vi "Create GB 2014-11-10.vi"(6 "Edge Duplication Range":dbl=3.0, 7 "Skip cleanup if no subset":bool, 8 "Reduce to Repeating":T2={"Slab X"=4.0, "Slab Y"=4.0, "Tolerance (A)"=0.5, "Presorted?"=FALSE}, 9 "Min Seperation Distance (A)":dbl=1.5, 10 "Grain Growth and Geometry":T3={"Grain 1 Length (prop)"=1.0, "Grain 2 Length (prop)"=1.0, "Max Grain Height (A)"=80.0, "Max Grain Width (A)"=80.0, "Grain 1 Start"=-0.001, "Overlap Region (A)"=0.001}, 11 "Grain Boundary Definition":T4={"Grain 1 Orientation"=[1.0, 1.0, 1.0], "Grain 2 Orientation"=[1.0, 1.0, 1.0], "Twist Angle (Deg)"=60.0, "Translation Vector"=[0.0, 0.0, 0.0]}) -> (0 "GB Data":string[][](array[string]), 1 "Reduced Orthorhombic?":bool=TRUE, 2 "Reduced Monoclinic?":bool=TRUE, 3 "Grain Boundary":T5={"Structure Name"="(60.0) twist [1,1,1] [1,1,1+0.0tilt] (0.00,0.00,0.00)T GB", "Lattice vector a"=[2.339033413721388, 4.05132471316672, 0.0], "Lattice vector b"=[4.678066827442776, 0.0, 0.0], "Lattice vector c"=[0.0, 0.0, 46.0], "Atoms Array"=[{"Atom Name"="Cd", "Positions (Direct)"=[[0.00024683284377352164, 9.034709130927474e-05, -0.0008722454374929306], [0.0002468328437733024, 9.034709130938435e-05, 0.24912775456250708], [0.0002468328437733024, 9.034709130938435e-05, 0.49912775456250713], [0.33358016617710656, 0.33342368042464277, 0.08305707760779221], [0.33358016617710656, 0.33342368042464277, 0.3321630930398645], [0.6669134995104397, 0.6667570137579764, 0.41519843151722197], [0.6669134995104399, 0.6667570137579764, 0.16609241608514966], [0.00024683284377352164, 9.034709130927474e-05, 0.749127754562507], [0.33358016617710673, 0.33342368042464277, 0.6660924160851497], [0.33358016617710695, 0.33342368042464265, 0.9151984315172218], [0.6669134995104401, 0.6667570137579764, 0.5830570776077922], [0.6669134995104403, 0.6667570137579764, 0.8321630930398645]], "Positions (Cartesian)"=[[0.0, 8.881784197001252e-16, -0.04112329012467342], [0.0, 0.0, 11.458876709875327], [0.0, 0.0, 22.958876709875327], [2.339033413721388, 1.350441571055573, 3.819625569958442], [2.339033413721388, 1.350441571055573, 15.278502279833768], [4.678066827442776, 2.700883142111145, 19.09812784979221], [4.678066827442776, 2.700883142111146, 7.639251139916884], [0.0, 8.881784197001252e-16, 34.45887670987533], [2.3390334137213884, 1.3504415710555737, 30.639251139916883], [2.3390334137213884, 1.3504415710555746, 42.098127849792206], [4.678066827442777, 2.700883142111147, 26.819625569958443], [4.678066827442777, 2.700883142111148, 38.278502279833766]]}, {"Atom Name"="Te", "Positions (Direct)"=[[0.0002468328437733024, 9.034709130938435e-05, 0.062298242988452865], [0.0002468328437733024, 9.034709130938435e-05, 0.31140425842052516], [0.3335801661771065, 0.33342368042464277, 0.14533358146581032], [0.3335801661771065, 0.33342368042464277, 0.39443959689788266], [0.6669134995104397, 0.6667570137579764, 0.47747493537524005], [0.6669134995104399, 0.6667570137579764, 0.22836891994316774], [0.000246832843773325, 9.034709130937305e-05, 0.5622982429884529], [0.00024683284377354425, 9.034709130926343e-05, 0.811404258420525], [0.33358016617710684, 0.3334236804246426, 0.7283689199431677], [0.33358016617710706, 0.3334236804246425, 0.97747493537524], [0.6669134995104401, 0.6667570137579764, 0.6453335814658103], [0.6669134995104403, 0.6667570137579764, 0.8944395968978825]], "Positions (Cartesian)"=[[0.0, 0.0, 2.864719177468832], [0.0, 0.0, 14.323595887344158], [2.339033413721388, 1.3504415710555728, 6.684344747427275], [2.339033413721388, 1.3504415710555728, 18.1432214573026], [4.678066827442776, 2.700883142111145, 21.96284702726104], [4.678066827442776, 2.700883142111146, 10.503970317385717], [0.0, 9.181246808733296e-17, 25.86471917746883], [0.0, 9.799908877874582e-16, 37.323595887344155], [2.339033413721388, 1.3504415710555742, 33.503970317385715], [2.339033413721388, 1.350441571055575, 44.96284702726104], [4.678066827442777, 2.700883142111147, 29.684344747427275], [4.678066827442777, 2.700883142111148, 41.1432214573026]]}], "# of atoms"=24} {"Atoms Array"."Positions (Cartesian)" format="%#_4f"; "Atoms Array"."Positions (Direct)" format="%#_4f"}, 4 "Creation Time":T1={"Time to create primitives"=0, "Time to Grow to Box"=52, "Time to find subset"=55, "Time to Cleanup"=10})   [LabVIEW 2010]
uses:
  <vilib>/Analysis/NI_AALPro.lvlib
  <vilib>/Analysis/_algsub.llb/Real Vector Norm.vi
  <vilib>/Analysis/NI_AALBase.lvlib
  <vilib>/Analysis/baseanly.llb/Real A x B.vi
  <vilib>/Analysis/baseanly.llb/A x Vector.vi
panel:
  in  "Headers":string[](array[string])=["Grain 1, h", "Grain 1, k", "Grain 1, L", "Grain 2, h", "Grain 2, k", "Grain 2, L", "Twist Angle (Deg)", "Translation Tx", "Translation Ty", "Translation Tz", "Tilt Angle (Deg)", "Viewing Angle, h", "Viewing Angle, k", "Viewing Angle, L", "Grain 1 Length (factor)", "Grain 2 Length (factor", "Max Grain Height (A)", "Max Grain Width (A)", "Grain 1 Start", "Overlap Region (A)", "Reduction Slab X", "Reduction Slab Y", "Reduction Tolerance (A)", "Min Atomic Separation Distance", "Edge Duplication Range", "# Atoms"]
  out "Monoclinic Atoms":i32
  out "Orthorhombic atoms":i32
  out "Time to Cleanup":u32=10
  out "Time to find subset":u32=55
  out "Time to Grow to Box":u32=52
  out "Time to create primitives":u32
  out "Tilt Angle":dbl
  out "# of Atoms Removed":i32=2
  out "Repeating Y Length Scale":dbl=8.10264942633344
  out "Repeating X Length Scale":dbl=4.678066827442776
  out "Mutual Viewing Angle":dbl[](array[numeric])=[1.0, -1.0, 0.0]
  in  "Conventional Unit Cell":T5={"Structure Name"="CdTe", "Lattice vector a"=[6.615785553057252, 0.0, 0.0], "Lattice vector b"=[0.0, 6.615785553057252, 0.0], "Lattice vector c"=[0.0, 0.0, 6.615785553057252], "Atoms Array"=[{"Atom Name"="Cd", "Positions (Direct)"=[[0.0, 0.0, 0.0], [0.0, 0.5, 0.5], [0.5, 0.0, 0.5], [0.5, 0.5, 0.0]], "Positions (Cartesian)"=[[0.0, 0.0, 0.0], [0.0, 3.307892776528626, 3.307892776528626], [3.307892776528626, 0.0, 3.307892776528626], [3.307892776528626, 3.307892776528626, 0.0]]}, {"Atom Name"="Te", "Positions (Direct)"=[[0.25, 0.25, 0.25], [0.75, 0.75, 0.25], [0.75, 0.25, 0.75], [0.25, 0.75, 0.75]], "Positions (Cartesian)"=[[1.653946388264313, 1.653946388264313, 1.653946388264313], [4.96183916479294, 4.96183916479294, 1.653946388264313], [4.96183916479294, 1.653946388264313, 4.96183916479294], [1.653946388264313, 4.96183916479294, 4.96183916479294]]}], "# of atoms"=8}
  # "Primitives"
  # "Grain Growth"
  # "Remove Collisions"
  # "Make into repeating cell"
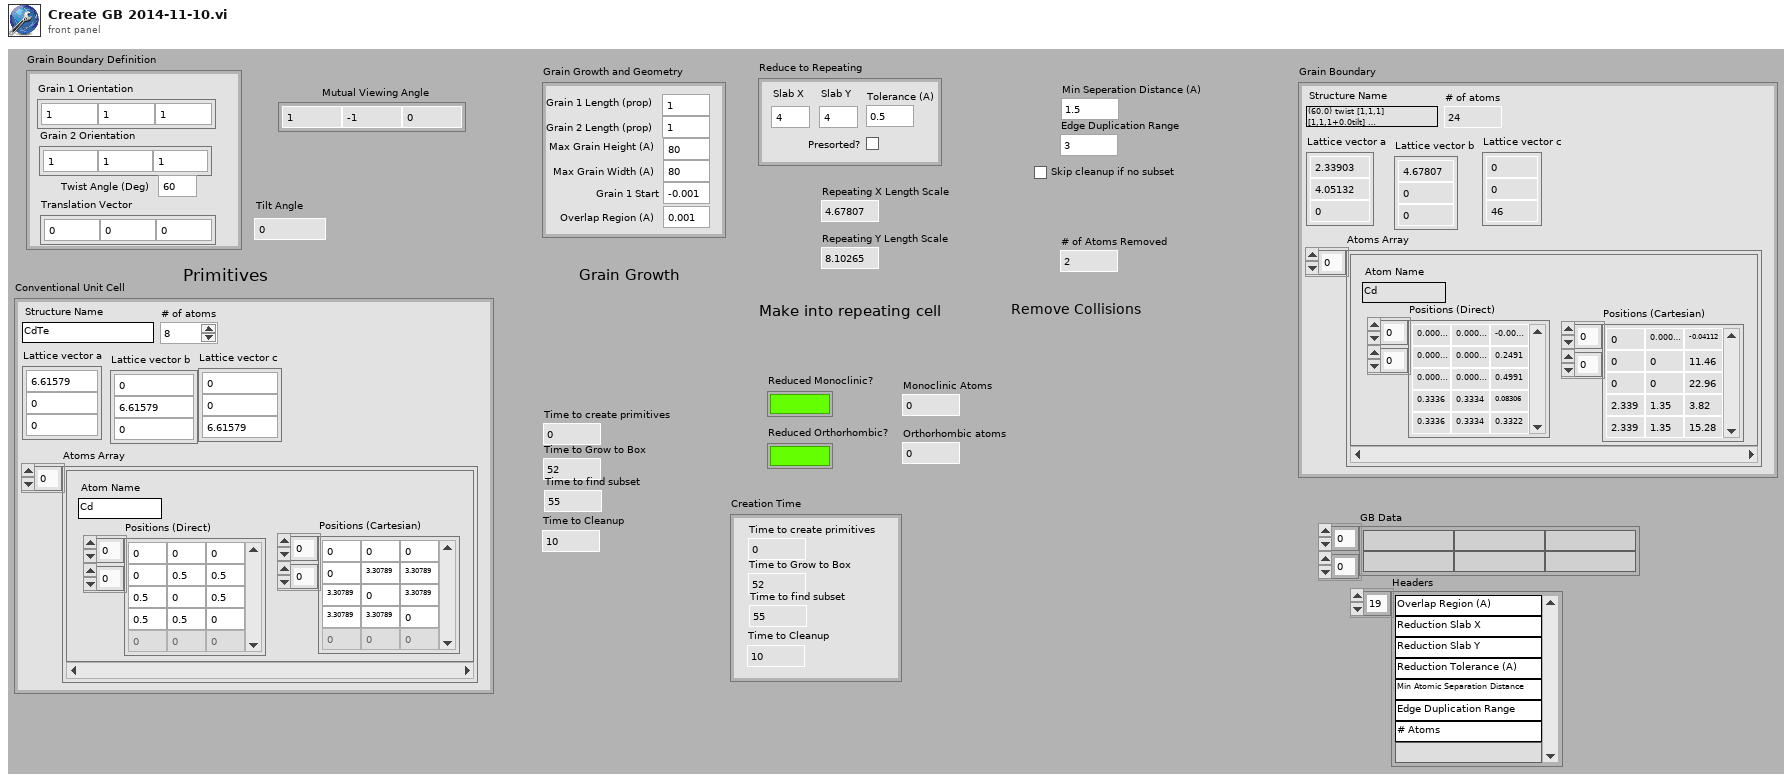
[diagram p1: front panel]
types:
  T1 = cluster{"Time to create primitives":u32, "Time to Grow to Box":u32, "Time to find subset":u32, "Time to Cleanup":u32}
  T2 = cluster{"Slab X":dbl, "Slab Y":dbl, "Tolerance (A)":dbl, "Presorted?":bool}
  T3 = cluster{"Grain 1 Length (prop)":dbl, "Grain 2 Length (prop)":dbl, "Max Grain Height (A)":dbl, "Max Grain Width (A)":dbl, "Grain 1 Start":dbl, "Overlap Region (A)":dbl}
  T4 = cluster{"Grain 1 Orientation":dbl[], "Grain 2 Orientation":dbl[], "Twist Angle (Deg)":dbl, "Translation Vector":dbl[]}
  T5 = cluster{"Structure Name":string, "Lattice vector a":dbl[], "Lattice vector b":dbl[], "Lattice vector c":dbl[], "Atoms Array":cluster{"Atom Name":string, "Positions (Direct)":dbl[][], "Positions (Cartesian)":dbl[][]}[], "# of atoms":i32}
  T6 = typedef "NI_Matrix.lvlib/RealMatrix.ctl" = dbl[][]
  T7 = cluster{"Z Min":dbl, "Max Grain Width (A)":dbl, "Z Min":dbl, "Max Grain Height (A)":dbl, "Grain 1 Start":dbl, dbl}
  T8 = cluster{"Grain 1 Start":dbl, "Max Grain Width (A)":dbl, "Grain 1 Start":dbl, "Max Grain Height (A)":dbl, dbl, dbl}
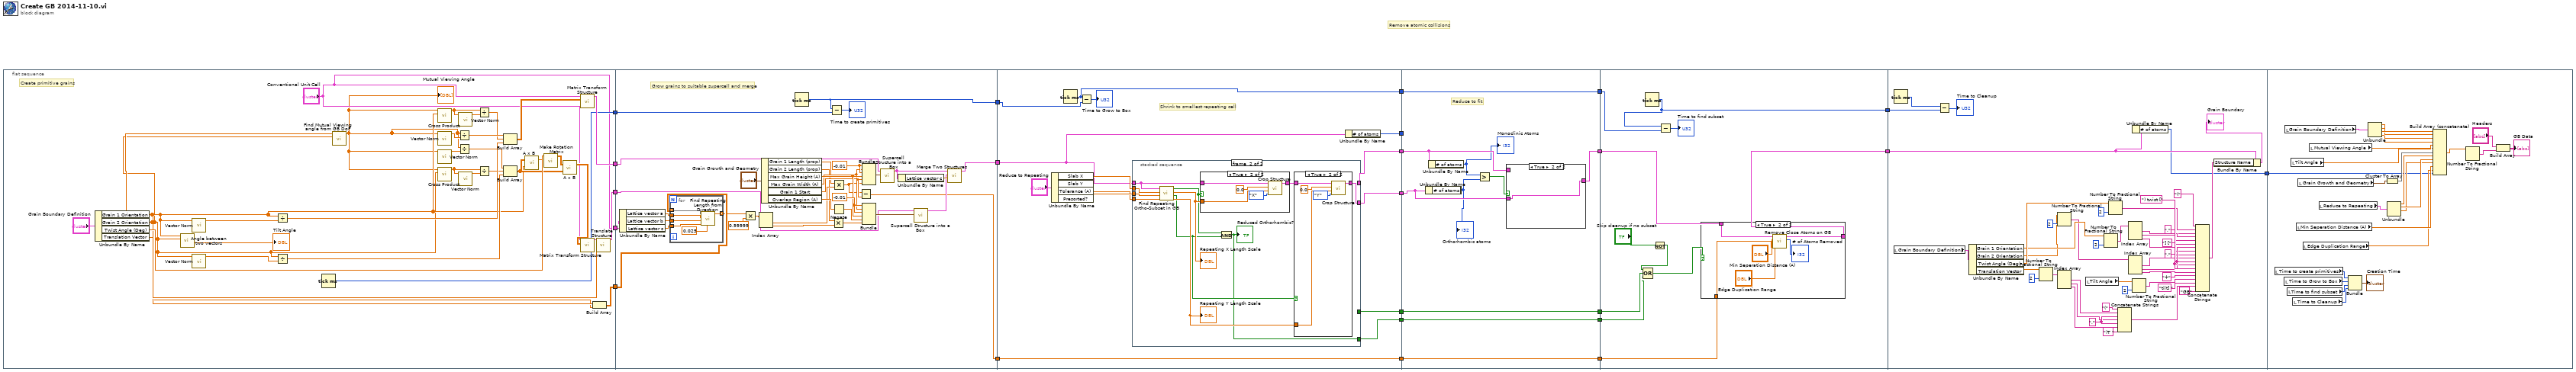
[diagram p0: block diagram]
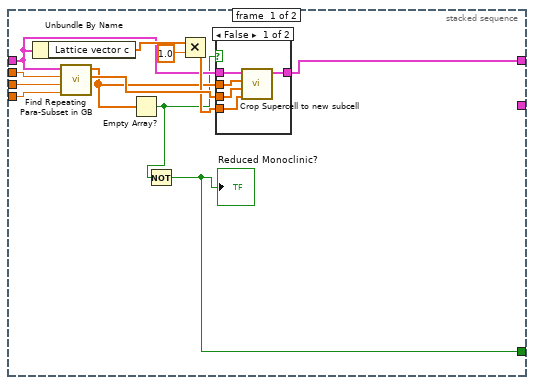
[diagram p2: hidden frame]
diagram:
  # "Remove atomic collisions"
  n1 = flat-sequence {
    tunnel: [w36] -> w23
    tunnel: [w47] -> w22
    tunnel: [w31] -> w19
    tunnel: ["Conventional Unit Cell"] -> w7
    tunnel: [w29] -> w6
    tunnel: w23 -> [w83]
    tunnel: w22 -> [w87]
    tunnel: [w79] -> w20
    tunnel: w19 -> [w73]
    tunnel: [w72] -> w18
    tunnel: [w70] -> w16
    tunnel: w7 -> [w69]
    tunnel: w6 -> [w65]
    tunnel: w20 -> [w99]
    tunnel: [w101] -> w15
    tunnel: w18 -> [w108]
    tunnel: [w106] -> w13
    tunnel: w16 -> [w105]
    tunnel: [w105] -> w11
    tunnel: [w100] -> w9
    tunnel: [w98] -> w8
    tunnel: [w97] -> w4
    tunnel: [w96] -> w3
    tunnel: w15 -> [w157]
    tunnel: [w155] -> w14
    tunnel: w13 -> [w160]
    tunnel: [w160] -> w12
    tunnel: w11 -> [w159]
    tunnel: [w159] -> w10
    tunnel: w9 -> [w156]
    tunnel: w8 -> [_]
    tunnel: w4 -> [w151]
    tunnel: w3 -> [w152]
    tunnel: [w152] -> w2
    tunnel: [w151] -> w1
    tunnel: w14 -> [w173]
    tunnel: [w172] -> w21
    tunnel: w12 -> [w170]
    tunnel: [w169] -> w17
    tunnel: w10 -> [w167]
    tunnel: w2 -> [w164]
    tunnel: w1 -> [w163]
    tunnel: w21 -> [w189]
    tunnel: w17 -> [w190]
    tunnel: [w188] -> w5
    tunnel: w5 -> [w236]
    frame #0 {
      # "Create primitive grains"
      n2 = Unbundle By Name("Grain Boundary Definition") -> ("Grain 1 Orientation"=w26:dbl[], "Grain 2 Orientation"=w25:dbl[], "Twist Angle (Deg)"=w33:dbl, "Translation Vector"=w32:dbl[])
      n3 = call "Angle between two vectors.vi"("Vector 2"=w25, "Vector 1"=w26) -> ("Angle (Degrees)"=→"Tilt Angle":dbl)  [unwired: 7 in, 2 out]
      n4 = call-poly <vilib>:"Vector Norm.vi"("Input Vector"=w26) -> ("norm"=w53:dbl)  [unwired: 9 in, 1 out]
      n5 = call-poly <vilib>:"Vector Norm.vi"("Input Vector"=w25) -> ("norm"=w39:dbl)  [unwired: 9 in, 1 out]
      n6 = Divide(x=w26, y=w53) -> (x/y=w51:dbl[])
      n7 = Divide(x=w25, y=w39) -> (x/y=w41:dbl[])
      n8 = Tick Count (ms)() -> (millisecond timer value=w31:u32)
      n9 = call "Find Mutual Viewing angle from GB DoF.vi"("Viewing Angle Tolerance (Deg)"=w25, "Grain Boundary Macro DoF"=w26) -> ("Mutual Viewing Angle"=w24:dbl[])  [unwired: 7 in, 2 out]
      "Mutual Viewing Angle" <- w24
      n10 = call <vilib>:"Cross Product.vi"("B Vector"=w26, "A Vector"=w24) -> ("Cross Product"=w49:dbl[])  [unwired: 8 in, 1 out]
      n11 = call-poly <vilib>:"Vector Norm.vi"("Input Vector"=w24) -> ("norm"=w55:dbl)  [unwired: 9 in, 1 out]
      n12 = call-poly <vilib>:"Vector Norm.vi"("Input Vector"=w24) -> ("norm"=w37:dbl)  [unwired: 9 in, 1 out]
      n13 = call <vilib>:"Cross Product.vi"("B Vector"=w25, "A Vector"=w24) -> ("Cross Product"=w42:dbl[])  [unwired: 8 in, 1 out]
      n14 = Divide(x=w24, y=w55) -> (x/y=w52:dbl[])
      n15 = Divide(x=w24, y=w37) -> (x/y=w40:dbl[])
      n16 = call-poly <vilib>:"Vector Norm.vi"("Input Vector"=w49) -> ("norm"=w54:dbl)  [unwired: 9 in, 1 out]
      n17 = call-poly <vilib>:"Vector Norm.vi"("Input Vector"=w42) -> ("norm"=w38:dbl)  [unwired: 9 in, 1 out]
      n18 = Divide(x=w49, y=w54) -> (x/y=w48:dbl[])
      n19 = Divide(x=w42, y=w38) -> (x/y=w46:dbl[])
      n20 = Build Array(w52, w48, w51) -> (w50:T6)
      n21 = Build Array(w40, w46, w41) -> (w28:T6)
      n22 = call-poly <vilib>:"A x B.vi"("Vector"=w26, "A"=w28) -> ("A x Vector"=w27:dbl[])  [unwired: 1 out]
      n23 = call "Make Rotation Matrix.vi"("Rotation Axis"=w27, "Rotation Angle (Degree)"=w33) -> ("Rotation Matrix"=w44:T6)  [unwired: 9 in]
      n24 = call-poly <vilib>:"A x B.vi"("B"=w28, "A"=w44) -> ("A x B"=w43:T6)  [unwired: 1 out]
      n25 = call "Matrix Transform Structure.vi"("Matrix Transform"=w50, "Original Structure"="Conventional Unit Cell") -> ("After Transform"=w47:T5)  [unwired: 9 in]
      n26 = call "Matrix Transform Structure.vi"("Matrix Transform"=w43, "Original Structure"="Conventional Unit Cell") -> ("After Transform"=w45:T5)  [unwired: 9 in]
      n27 = Build Array(w26, w25) -> (w29:dbl[][])
      n28 = call "Translate Structure.vi"("Translation Vector (Cartesian)"=w32, "Atomic Structure"=w45) -> ("Shifted Structure"=w36:T5)  [unwired: 9 in]
    }
    frame #1 {
      w86 = -0.01 ("Z Min")
      w89 = -0.01 ("Grain 1 Start")
      # "Grow grains to suitable supercell and merge"
      n29 = Unbundle By Name(w69) -> ("Lattice vector a"=w68:dbl[], "Lattice vector b"=w67:dbl[], "Lattice vector c"=w66:dbl[])
      n30 = for {
        tunnel: w68 -> [w95]
        tunnel: w67 -> [w94]
        tunnel: w66 -> [w93]
        tunnel: [w91] -> w57 mode=indexing
        tunnel: w65 -> [w90] mode=indexing
        n31 = call "Find Repeating Length from Direction.vi"("Tolerance"=0.025, "Lattice vector c"=w93, "Lattice vector b"=w94, "Lattice vector a"=w95, "Direction"=w90) -> ("Repeating Length (A)"=w91:dbl)  [unwired: 6 in]
      }
      n32 = Multiply(x=w57, y=0.99999) -> (x*y=w56:dbl[])
      n33 = Index Array(array=w56) -> (element #1=w63:dbl, element #2=w60:dbl)  [unwired: 2 in]
      n34 = Unbundle By Name("Grain Growth and Geometry") -> ("Grain 1 Length (prop)"=w64:dbl, "Grain 2 Length (prop)"=w61:dbl, "Max Grain Height (A)"=w76:dbl, "Max Grain Width (A)"=w75:dbl, "Grain 1 Start"=w71:dbl, "Overlap Region (A)"=w77:dbl)
      n35 = Tick Count (ms)() -> (millisecond timer value=w72:u32)
      n36 = Subtract(x=w72, y=w73) -> (x-y=→"Time to create primitives":u32)
      n37 = Multiply(x=w61, y=w60) -> (x*y=w59:dbl)
      n38 = Multiply(x=w64, y=w63) -> (x*y=w62:dbl)
      n39 = Negate(x=w77) -> (-x=w88:dbl)
      n40 = Subtract(x=w62, y=w71) -> (x-y=w70:dbl)
      n41 = Bundle("Z Min"=w86, "Max Grain Width (A)"=w75, "Z Min"=w86, "Max Grain Height (A)"=w76, "Grain 1 Start"=w71, w62) -> (w85:T7)  [unwired: 1 in]
      n42 = Bundle("Grain 1 Start"=w89, "Max Grain Width (A)"=w75, "Grain 1 Start"=w89, "Max Grain Height (A)"=w76, w88, w59) -> (w84:T8)  [unwired: 1 in]
      n43 = call "Supercell Structure into a Box.vi"("Draw Box"=w85, "Subcrystal"=w87) -> ("Expanded cubic Structure"=w80:T5)  [unwired: 7 in, 2 out]
      n44 = Unbundle By Name(w80) -> ("Lattice vector c"=w82:dbl[])
      n45 = call "Supercell Structure into a Box.vi"("Draw Box"=w84, "Subcrystal"=w83) -> ("Expanded cubic Structure"=w81:T5)  [unwired: 7 in, 2 out]
      n46 = call "Merge Two Structures.vi"("Translation Vector (1 to 2)"=w82, "Atomic Structure 2"=w81, "Atomic Structure 1"=w80) -> ("Atomic Structure of 1 + 2 by T"=w79:T5)  [unwired: 8 in]
    }
    frame #2 {
      # "Shrink to smallest repeating cell"
      n47 = Unbundle By Name("Reduce to Repeating") -> ("Slab X"=w104:dbl, "Slab Y"=w103:dbl, "Tolerance (A)"=w102:dbl)  [unwired: 1 out]
      n48 = Tick Count (ms)() -> (millisecond timer value=w106:u32)
      n49 = Subtract(x=w106, y=w108) -> (x-y=→"Time to Grow to Box":u32)
      n50 = stacked-sequence {
        tunnel: [w113 _] -> w101
        tunnel: w104 -> [w116 w138]
        tunnel: w103 -> [w115 w137]
        tunnel: w102 -> [w114 w136]
        tunnel: w99 -> [w117 w135]
        tunnel: [_ w131] -> w100
        tunnel: [_ w128] -> w97
        tunnel: [w110 _] -> w96
        frame #0 {
          n51 = Unbundle By Name(w117) -> ("Lattice vector c"=w119:dbl[])
          n52 = call "Find Repeating Para-Subset in GB.vi"("Tolerance (A)"=w114, "Slab Y"=w115, "Slab X"=w116, "Supercell Structure"=w117) -> ("New Lattice Vector b"=w121:dbl[], "New Lattice Vector a"=w112:dbl[])  [unwired: 5 in, 1 out]
          n53 = Empty Array?(array=w112) -> (empty?=w111:bool)
          n54 = Not(x=w111) -> (.not. x?=w110:bool)
          "Reduced Monoclinic?" <- w110
          n55 = Multiply(x=w119, y=1.0) -> (x*y=w118:dbl[])
          n56 = case shown="False" w111 {
            tunnel: w121 -> [w126 _]
            tunnel: w112 -> [w125 _]
            tunnel: w118 -> [w124 _]
            tunnel: w117 -> [w123 w127]
            tunnel: [w122 w127] -> w113
            frame False {
              n57 = call "Crop Supercell to new subcell.vi"("New Lattice Vector c"=w124, "New Lattice Vector b"=w126, "New Lattice Vector a"=w125, "Supercell Structure"=w123) -> ("Reduced Structure"=w122:T5)  [unwired: 7 in]
            }
            frame True {
            }
          }
        }
        frame #1 {
          n58 = call "Find Repeating Ortho-Subset in GB.vi"("Tolerance (A)"=w136, "Slab Y"=w137, "Slab X"=w138, "Grain Boundary"=w135) -> ("Repeating Y Length Scale"=w132:dbl, "Subset Y found?!"=w129:bool, "Repeating X Length Scale"=w133:dbl, "Subset X found?!"=w130:bool)  [unwired: 4 in]
          "Repeating X Length Scale" <- w133
          "Repeating Y Length Scale" <- w132
          n59 = case shown="True" w130 {
            tunnel: w135 -> [w145 w150]
            tunnel: [w145 w147] -> w134
            tunnel: w133 -> [_ w146]
            frame False {
            }
            frame True {
              n60 = call "Crop Structure.vi"("Cropping Index"=enum16{"X", "Y", "Z"}."X", "Upper Bound Z"=w146, "Lower bound Z"=0.0, "Input Structure"=w150) -> ("Cropped Structure"=w147:T5)  [unwired: 7 in]
            }
          }
          n61 = And(x=w130, y=w129) -> (x .and. y?=w128:bool)
          "Reduced Orthorhombic?" <- w128
          n62 = case shown="True" w129 {
            tunnel: w134 -> [w139 w144]
            tunnel: w132 -> [_ w142]
            tunnel: [w139 w140] -> w131
            frame False {
            }
            frame True {
              n63 = call "Crop Structure.vi"("Cropping Index"=enum16{"X", "Y", "Z"}."Y", "Upper Bound Z"=w142, "Lower bound Z"=0.0, "Input Structure"=w144) -> ("Cropped Structure"=w140:T5)  [unwired: 7 in]
            }
          }
        }
      }
      n64 = Unbundle By Name(w99) -> ("# of atoms"=w98:i32)
    }
    frame #3 {
      # "Reduce to fit"
      n65 = Unbundle By Name(w156) -> ("# of atoms"=w153:i32)
      "Orthorhombic atoms" <- w153
      n66 = Unbundle By Name(w157) -> ("# of atoms"=w154:i32)
      "Monoclinic Atoms" <- w154
      n67 = Greater?(x=w154, y=w153) -> (0:w158:bool)
      n68 = case shown="True" w158 {
        tunnel: [w161 w162] -> w155
        tunnel: w157 -> [w161 _]
        tunnel: w156 -> [_ w162]
        frame False {
        }
        frame True {
        }
      }
    }
    frame #4 {
      n69 = Tick Count (ms)() -> (millisecond timer value=w169:u32)
      n70 = Not(x="Skip cleanup if no subset") -> (.not. x?=w166:bool)
      n71 = Compound Arithmetic op=OR(w166, w164, w163) -> (w165:bool)
      n72 = Subtract(x=w169, y=w170) -> (x-y=→"Time to find subset":u32)
      n73 = case shown="True" w165 {
        tunnel: w173 -> [w174 w178]
        tunnel: [w174 w177] -> w172
        tunnel: w167 -> [_ w175]
        frame False {
        }
        frame True {
          n74 = call "Remove Close Atoms on GB.vi"("Grain Boundary Location (A)"=w175, "Edge Duplication Range"="Edge Duplication Range", "Minimally Allowable Distance (A)"="Min Seperation Distance (A)", "Structure"=w178) -> ("# of Atoms Removed"=→"# of Atoms Removed":i32, "Structure with atoms removed"=w177:T5)  [unwired: 6 in]
        }
      }
    }
    frame #5 {
      w216 = "," ("string")
      w205 = "," ("string")
      n75 = local read "Grain Boundary Definition"() -> (w221:T4)
      n76 = Tick Count (ms)() -> (millisecond timer value=w191:u32)
      n77 = Subtract(x=w191, y=w190) -> (x-y=→"Time to Cleanup":u32)
      n78 = Unbundle By Name(w221) -> ("Grain 1 Orientation"=w185:dbl[], "Grain 2 Orientation"=w182:dbl[], "Twist Angle (Deg)"=w222:dbl, "Translation Vector"=w223:dbl[])
      n79 = Number To Fractional String(number=w223, precision (6)=i16 2) -> (F-format string=w212:string[])  [unwired: 2 in]
      n80 = Number To Fractional String(number=w182, precision (6)=i16 2) -> (F-format string=w181:string[])  [unwired: 2 in]
      n81 = Index Array(array=w212) -> (element #1=w213:string, element #2=w215:string, element #3=w217:string)  [unwired: 3 in]
      n82 = local read "Tilt Angle"() -> (w224:dbl)
      n83 = Number To Fractional String(number=w185, precision (6)=i16 2) -> (F-format string=w184:string[])  [unwired: 2 in]
      n84 = Number To Fractional String(number=w222, precision (6)=i16 2) -> (F-format string=w196:string)  [unwired: 2 in]
      n85 = Concatenate Strings("(" ("string"), w213, w216, w215, w216, w217, ")T " ("string")) -> (w219:string)
      n86 = Index Array(array=w184) -> (element #1=w198:string, element #2=w200:string, element #3=w201:string)  [unwired: 3 in]
      n87 = Index Array(array=w181) -> (element #1=w203:string, element #2=w204:string, element #3=w206:string)  [unwired: 3 in]
      n88 = Unbundle By Name(w189) -> ("# of atoms"=w188:i32)
      n89 = Number To Fractional String(number=w224, precision (6)=i16 2) -> (F-format string=w208:string)  [unwired: 2 in]
      n90 = Concatenate Strings("(" ("string"), w196, ") twist [" ("string"), w198, "," ("string"), w200, w205, w201, "] [" ("string"), w203, w205, w204, w205, w206, "+" ("string"), w208, "tilt] " ("string"), w219, "GB" ("string")) -> (w193:string)
      n91 = Bundle By Name(cluster=w189, "Structure Name"=w193) -> (→"Grain Boundary":T5)
    }
    frame #6 {
      n92 = local read "Time to create primitives"() -> (w228:u32)
      n93 = local read "Time to Grow to Box"() -> (w227:u32)
      n94 = local read "Grain Boundary Definition"() -> (w249:T4)
      n95 = local read "Time to find subset"() -> (w226:u32)
      n96 = local read "Tilt Angle"() -> (w232:dbl)
      n97 = local read "Time to Cleanup"() -> (w229:u32)
      n98 = local read "Min Seperation Distance (A)"() -> (w238:dbl)
      n99 = local read "Grain Growth and Geometry"() -> (w244:T3)
      n100 = local read "Edge Duplication Range"() -> (w237:dbl)
      n101 = local read "Mutual Viewing Angle"() -> (w231:dbl[])
      n102 = local read "Reduce to Repeating"() -> (w242:T2)
      n103 = Bundle("Time to create primitives"=w228, "Time to Grow to Box"=w227, "Time to find subset"=w226, "Time to Cleanup"=w229) -> (→"Creation Time":T1)  [unwired: 1 in]
      n104 = Unbundle(w249) -> ("Grain 1 Orientation"=w248:dbl[], "Grain 2 Orientation"=w247:dbl[], "Twist Angle (Deg)"=w246:dbl, "Translation Vector"=w245:dbl[])
      n105 = Cluster To Array(cluster=w244) -> (array=w243:dbl[])
      n106 = Unbundle(w242) -> ("Slab X"=w241:dbl, "Slab Y"=w240:dbl, "Tolerance (A)"=w239:dbl)  [unwired: 1 out]
      n107 = Build Array (concatenate)(w248, w247, w246, w245, w232, w231, w243, w241, w240, w239, w238, w237, w236) -> (w235:dbl[])
      n108 = Number To Fractional String(number=w235) -> (F-format string=w234:string[])  [unwired: 3 in]
      n109 = Build Array("Headers", w234) -> (→"GB Data":string[][])
    }
  }
